vi "Start Cam Cal.vi"(8 "error in (no error)":errorcluster, 11 "main gui queue":refnum<queue>) -> (0 "error out":errorcluster)   [LabVIEW 2020]
uses:
  GUI/Main GUI Loop/Handler.ctl
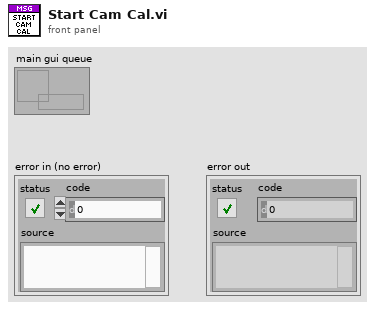
[diagram p1: front panel]
types:
  T1 = typedef "Handler.ctl" = cluster{"bool ref":refnum<vi>, "error":errorcluster, "msg":string, "status":string, "switch status":bool, "force cal":dbl[][], "force cal results":dbl[][]}
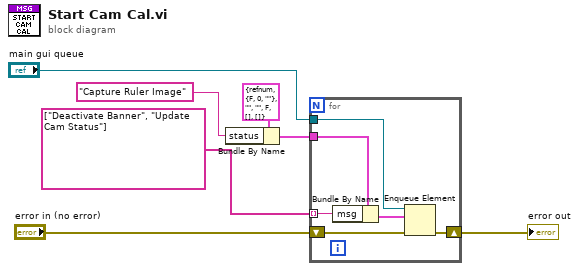
[diagram p0: block diagram]
diagram:
  n1 = Bundle By Name(cluster=T1 {"bool ref"=refnum, "error"={"status"=FALSE, "code"=0, "source"=""}, "msg"="", "status"="", "switch status"=FALSE, "force cal"=[], "force cal results"=[]} ("main gui type"), "status"="Capture Ruler Image") -> (w4:T1)
  n2 = for {
    shift-right: [w12] -> w1
    shift-left: "error in (no error)" -> [w13]
    tunnel: string[] ["Deactivate Banner", "Update Cam Status"] ("msg") -> [w11] mode=indexing
    tunnel: w4 -> [w10]
    tunnel: "main gui queue" -> [w9]
    n3 = Bundle By Name(cluster=w10, "msg"=w11) -> (w8:T1)
    n4 = Enqueue Element(queue=w9, element=w8, error in (no error)=w13) -> (error out=w12:errorcluster)  [unwired: 1 in, 2 out]
  }
  "error out" <- w1
